vi "STSatZ_v2.vi"() -> ()   [LabVIEW 2014]
uses:
  shared/CorrelImages (SubVI)Single.vi
  <userlib>/Nanonis Prog Interface V5/Nanonis Prog Interface.lvlib
panel:
  in  "Initial STS bias (V)":sgl format="%#_5p"
  in  "Ref Bias (V)":sgl=-0.4 format="%_2p"
  in  "Ref Current":sgl=3e-10 format="%#_6p"
  out "y drift":sgl format="%#_3p"
  out "x drift":sgl format="%#_3p"
  in  "DC every points":i32=1
  out "DC active":bool=TRUE
  out "Points taken":i32
  in  "PLL (F=OFF)":bool=TRUE
  in  "DC On":bool=TRUE
  in  "Channel index (0-23)":u8(ring) items=["Current"=0, "Z (m)"=14]
  in  "Img Speed":sgl=3e-08 format="%#_6p"
  in  "Img Bias (V)":sgl=0.02 format="%_2p"
  in  "Img Current":sgl=5e-12 format="%#_6p"
  in  "Drift correction Pixels":i32=256
  in  "Ref Tip Offset":dbl format="%#_6p"
  in  "movement delay (ms)":u32=750
  in  "setpoint delay (ms)":u32=750
  in  "z step":dbl=5e-11 format="%#_6p"
  in  "z range":dbl=4e-10 format="%#_6p"
  out "points":i32=9
  # "Draw Ref point as a marker"
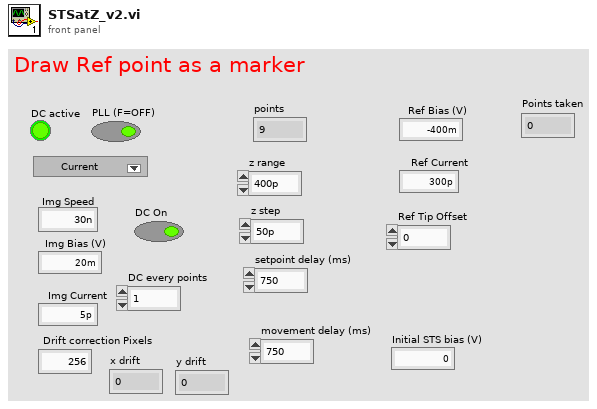
[diagram p1: front panel]
types:
  T1 = cluster{"X (m)":sgl, "Y (m)":sgl, "Text":string, "Color":u32, "Visible":bool}[]
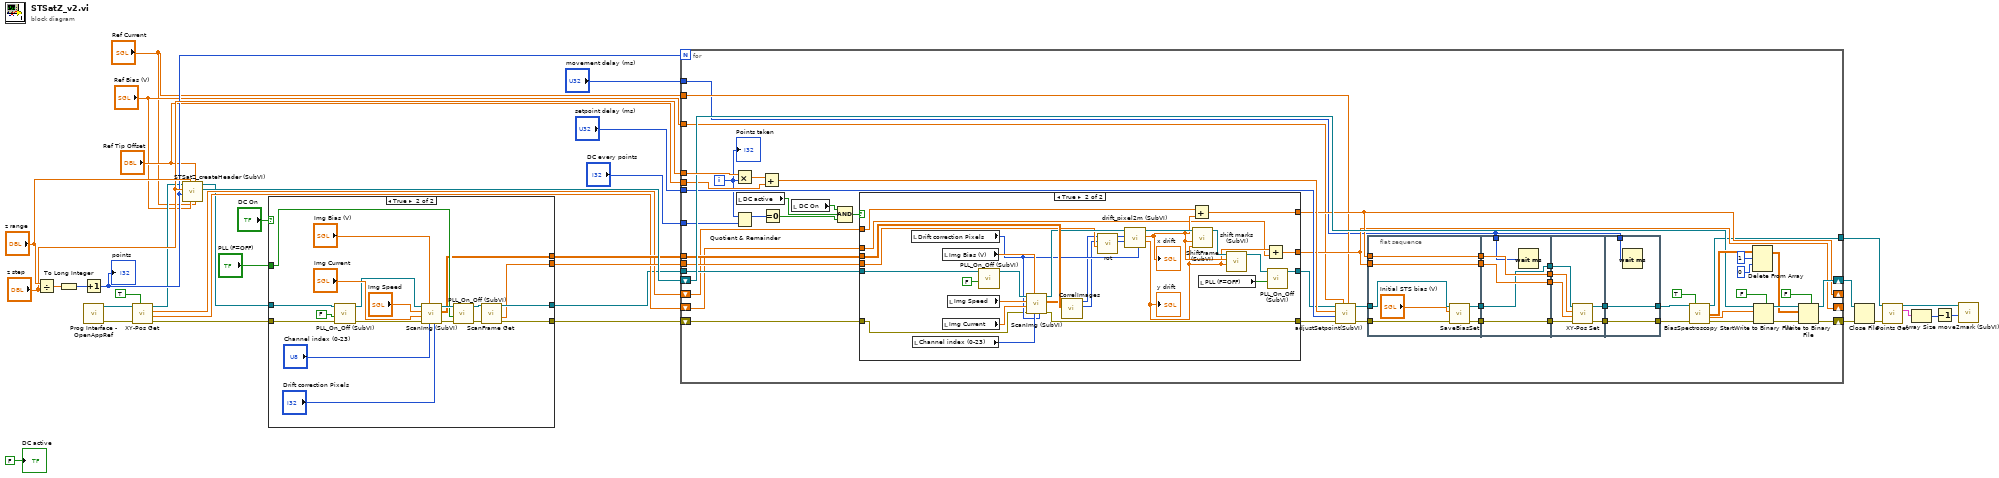
[diagram p0: block diagram]
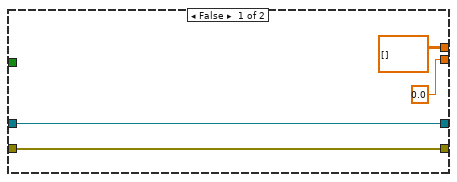
[diagram p2: hidden frame]
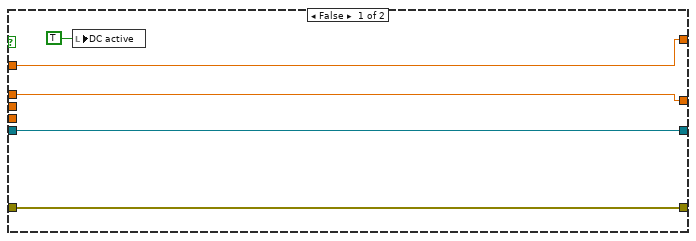
[diagram p3: hidden frame]
diagram:
  n1 = Divide(x="z range", y="z step") -> (x/y=w35:dbl)
  n2 = To Long Integer(number=w35) -> (32bit integer=w7:i32)
  n3 = Increment(x=w7) -> (x+1=w28:i32)
  "points" <- w28
  n4 = call <userlib>:"Prog Interface - OpenAppRef.vi"() -> ("Error out"=w19:errorcluster, "Application reference"=w20:refnum<vi>)  [unwired: 6 in]
  n5 = call <userlib>:"XY-Pos Get.vi"("Wait for newest data (F=False)"=TRUE, "error in (no error)"=w19, "Application ref in"=w20) -> ("error out"=w18:errorcluster, "Y (m)"=w17:sgl, "X (m)"=w16:sgl, "Application ref out"=w12:refnum<vi>)  [unwired: 4 in]
  n6 = call "STSatZ_createHeader (SubVI).vi"("Current"="Ref Current", "TipOffset"="Ref Tip Offset", "Bias"="Ref Bias (V)", "z range"="z range", "points"=w28, "z step"="z step", "Application in"=w12) -> ("File ref"=w34:refnum<file>, "Application out"=w11:refnum<vi>)  [unwired: 2 in, 1 out]
  n7 = case shown="True" "DC On" {
    tunnel: [w38 w46] -> w13
    tunnel: [w36 w45] -> w14
    tunnel: [sgl 0.0 ("Angle (deg)") w42] -> w23
    tunnel: w11 -> [w38 w44]
    tunnel: "PLL (F=OFF)" -> [_ w43]
    tunnel: [dbl[][] [] ("Img") w41] -> w24
    tunnel: w18 -> [w36 w40]
    frame False {
    }
    frame True {
      n8 = call "PLL_On_Off (SubVI).vi"("error in (no error)"=w40, "Output ON/OFF (F=OFF)"=FALSE, "Application in"=w44) -> ("error out"=w51:errorcluster, "Application out"=w52:refnum<vi>)  [unwired: 7 in]
      n9 = call "ScanImg (SubVI).vi"("pixel"="Drift correction Pixels", "Channel index (0-23)"="Channel index (0-23)", "Bias (V)"="Img Bias (V)", "error in (no error)"=w51, "Current"="Img Current", "Img Speed"="Img Speed", "Application in"=w52) -> ("error out"=w55:errorcluster, "Img"=w41:dbl[][], "Application out"=w56:refnum<vi>)  [unwired: 2 in]
      n10 = call "PLL_On_Off (SubVI).vi"("error in (no error)"=w55, "Output ON/OFF (F=OFF)"=w43, "Application in"=w56) -> ("error out"=w47:errorcluster, "Application out"=w48:refnum<vi>)  [unwired: 7 in]
      n11 = call <userlib>:"ScanFrame Get.vi"("Application ref in"=w48, "error in (no error)"=w47) -> ("Application ref out"=w46:refnum<vi>, "Angle (deg)"=w42:sgl, "error out"=w45:errorcluster)  [unwired: 9 in, 2 out]
    }
  }
  n12 = for {
    N: w28 -> [_]
    tunnel: "z step" -> [w112]
    tunnel: w13 -> [w85]
    shift-right: [w100] -> w33
    shift-left: w34 -> [w98]
    shift-right: [w99] -> w32
    shift-left: w14 -> [w83]
    tunnel: "setpoint delay (ms)" -> [w92]
    tunnel: "movement delay (ms)" -> [w61]
    tunnel: "Ref Tip Offset" -> [w88]
    tunnel: w24 -> [w81]
    tunnel: w23 -> [w80]
    tunnel: "DC every points" -> [w78]
    shift-right: [w73] -> _
    shift-left: w16 -> [w74]
    shift-right: [w71] -> _
    shift-left: w17 -> [w72]
    tunnel: "Ref Bias (V)" -> [w70]
    tunnel: "Ref Current" -> [w69]
    tunnel: [w59] -> w2
    i -> [w79]
    n13 = Multiply(x=w112, y=w79) -> (x*y=w97:dbl)
    n14 = Quotient & Remainder(x=w79, y=w78) -> (x-y*floor(x/y)=w77:i32)  [unwired: 1 out]
    n15 = local read "DC active"() -> (w87:bool)
    n16 = Add(x=w97, y=w88) -> (x+y=w89:dbl)
    n17 = Equal To 0?(x=w77) -> (x = 0?=w76:bool)
    n18 = local read "DC On"() -> (w86:bool)
    n19 = Compound Arithmetic op=AND(w86, w87, w76) -> (w75:bool)
    n20 = case shown="True" w75 {
      tunnel: w81 -> [_ w146]
      tunnel: w85 -> [w117 w137]
      tunnel: [w115 w145] -> w82
      tunnel: [w117 w135] -> w84
      tunnel: w80 -> [_ w132]
      tunnel: w83 -> [w115 w126]
      tunnel: [w114 w122] -> w73
      tunnel: w74 -> [w114 w123]
      tunnel: w72 -> [w113 w119]
      tunnel: [w113 w118] -> w71
      frame False {
        n21 = local write "DC active"(TRUE ("DC active")) -> ()
      }
      frame True {
        n22 = local read "Drift correction Pixels"() -> (w133:i32)
        n23 = local read "Channel index (0-23)"() -> (w140:u8)
        n24 = local read "Img Bias (V)"() -> (w141:sgl)
        n25 = local read "Img Current"() -> (w142:sgl)
        n26 = local read "Img Speed"() -> (w143:sgl)
        n27 = call "PLL_On_Off (SubVI).vi"("Output ON/OFF (F=OFF)"=FALSE, "Application in"=w137) -> ("Application out"=w136:refnum<vi>)  [unwired: 8 in, 1 out]
        n28 = call "ScanImg (SubVI).vi"("pixel"=w133, "Channel index (0-23)"=w140, "Bias (V)"=w141, "error in (no error)"=w126, "Current"=w142, "Img Speed"=w143, "Application in"=w136) -> ("error out"=w145:errorcluster, "Img"=w144:dbl[][], "Application out"=w138:refnum<vi>)  [unwired: 2 in]
        n29 = call-poly "CorrelImages.vi"("Ref Array"=w146, "New Image"=w144) -> ("Y drift"=w129:i32, "X drift"=w131:i32)  [unwired: 6 in, 2 out]
        n30 = call "rot.vi"("angle"=w132, "y"=w129, "x"=w131) -> ("y'"=w128:i32, "x'"=w130:i32)  [unwired: 7 in]
        n31 = call "drift_pixel2m (SubVI).vi"("Application in"=w138, "X drift"=w130, "Y drift"=w128, "Drift correction Pixels"=w133) -> ("Application out"=w139:refnum<vi>, "x drift"=w121:sgl, "y drift"=w120:sgl)  [unwired: 2 in, 1 out]
        "x drift" <- w121
        "y drift" <- w120
        n32 = Add(x=w123, y=w121) -> (x+y=w122:sgl)
        n33 = call "ShiftFrame (SubVI).vi"("Y shift"=w120, "X shift"=w121, "Application in"=w139) -> ("Application out"=w125:refnum<vi>)  [unwired: 8 in]
        n34 = local read "PLL (F=OFF)"() -> (w127:bool)
        n35 = call "shift marks (SubVI).vi"("y"=w120, "x"=w121, "Application in"=w125) -> ("Application out"=w124:refnum<vi>)  [unwired: 7 in, 1 out]
        n36 = Add(x=w120, y=w119) -> (x+y=w118:sgl)
        n37 = call "PLL_On_Off (SubVI).vi"("Output ON/OFF (F=OFF)"=w127, "Application in"=w124) -> ("Application out"=w135:refnum<vi>)  [unwired: 8 in, 1 out]
      }
    }
    n38 = call "adjustSetpoint(SubVI).vi"("Current"=w69, "Bias (V)"=w70, "error in (no error)"=w82, "milliseconds to wait"=w92, "tipLift"=w89, "Application in"=w84) -> ("error out"=w95:errorcluster, "Application out"=w96:refnum<vi>)  [unwired: 4 in]
    n39 = flat-sequence {
      tunnel: w71 -> [w152]
      tunnel: w73 -> [w153]
      tunnel: w95 -> [w151]
      tunnel: w96 -> [w147]
      tunnel: [w149] -> w67
      tunnel: [w153] -> w65
      tunnel: [w152] -> w63
      tunnel: [w150] -> w60
      tunnel: [w154] -> w68
      tunnel: w67 -> [w158]
      tunnel: [w158] -> w66
      tunnel: w65 -> [w157]
      tunnel: [w157] -> w64
      tunnel: w63 -> [w156]
      tunnel: [w156] -> w62
      tunnel: w61 -> [w155]
      tunnel: w60 -> [w154]
      tunnel: [w162] -> w91
      tunnel: [w161] -> w90
      tunnel: w68 -> [w164]
      tunnel: w66 -> [w163]
      tunnel: w64 -> [w160]
      tunnel: w62 -> [w159]
      tunnel: [w166] -> w93
      tunnel: [w167] -> w94
      tunnel: w91 -> [w167]
      tunnel: w90 -> [w166]
      tunnel: w61 -> [w165]
      frame #0 {
        n40 = call "SaveBiasSet.vi"("Application ref in"=w147, "Bias (V)"="Initial STS bias (V)", "error in (no error)"=w151) -> ("Application ref out"=w150:refnum<vi>, "Error out"=w149:errorcluster)  [unwired: 6 in]
      }
      frame #1 {
        n41 = Wait (ms)(milliseconds to wait=w155) -> ()  [unwired: 1 out]
      }
      frame #2 {
        n42 = call <userlib>:"XY-Pos Set.vi"("error in (no error)"=w163, "Y (m)"=w159, "X (m)"=w160, "Application ref in"=w164) -> ("error out"=w161:errorcluster, "Application ref out"=w162:refnum<vi>)  [unwired: 4 in]
      }
      frame #3 {
        n43 = Wait (ms)(milliseconds to wait=w165) -> ()  [unwired: 1 out]
      }
    }
    n44 = call <userlib>:"BiasSpectroscopy Start.vi"("Application ref in"=w94, "Get data (F)"=TRUE, "Error in (no error)"=w93) -> ("Application ref out"=w59:refnum<vi>, "Data"=w103:sgl[][], "Parameters"=w101:sgl[], "Error out"=w102:errorcluster)  [unwired: 8 in, 1 out]
    n45 = Delete From Array(array=w103, length=1, index (row)=0 ("index")) -> (array with subset deleted=w109:sgl[][])  [unwired: 1 in, 1 out]
    n46 = Write to Binary File(file (use dialog)=w98, data=w101, error in=w102, 5:FALSE ("prepend array or string size? (T)")) -> (refnum out=w110:refnum<file>, error out=w104:errorcluster)  [unwired: 2 in, 1 out]
    n47 = Write to Binary File(file (use dialog)=w110, data=w109, error in=w104, 5:FALSE ("prepend array or string size? (T)")) -> (refnum out=w100:refnum<file>, error out=w99:errorcluster)  [unwired: 2 in, 1 out]
    "Points taken" <- w79
  }
  n48 = Close File(refnum=w33, error in=w32) -> (error out=w1:errorcluster)  [unwired: 1 out]
  n49 = call <userlib>:"Points Get.vi"("Application ref in"=w2, "error in (no error)"=w1) -> ("Application ref out"=w3:refnum<vi>, "Points"=w6:T1)  [unwired: 11 in, 1 out]
  n50 = Array Size(array=w6) -> (size(s)=w5:i32)
  n51 = Decrement(x=w5) -> (x-1=w4:i32)
  n52 = call "move2mark (SubVI).vi"("index"=w4, "Application in"=w3) -> ()  [unwired: 9 in, 1 out]
  "DC active" <- FALSE ("DC active")
